vi "DSF.Memory.Pointer.Channel Properties.Write.1D.vi"(7 "count (-1: all)":i64=-1 format="%d elements", 8 "error in (no error)":errorcluster, 9 "buffer in":T1[](array[typedef]) {"count" format="%d elements"; "size" format="%d bytes"; "offset" format="%d bytes"}, 10 "index (0)":u64 format="%d elements", 11 "Channel Properties Pointer in":refnum<class "DSF.Memory.Pointer.Channel Properties.lvclass">) -> (0 "error out":errorcluster, 1 "buffer out":T1[](array[typedef]) {"count" format="%d elements"; "size" format="%d bytes"; "offset" format="%d bytes"}, 2 "index out":u64 format="%d elements", 3 "Channel Properties Pointer out":refnum<class "DSF.Memory.Pointer.Channel Properties.lvclass">)   [LabVIEW 2016, in "DSF.Memory.lvlib" / "DSF.Memory.Pointer.Channel Properties.lvclass"]
uses:
  DSF.Memory.Pointer.Channel Properties.lvclass
  C:/Git/SourceTree/DSF/Source/Classes/Memory.Pointer.Array/DSF.Memory.Pointer.Array.lvclass
  C:/Git/SourceTree/DSF/Source/Submodules/Memory Manager/Source/Classes/Pointer/Memory.Pointer.lvclass
  Typedefs/DSF.Common.Channel Configuration.ctl
  Typedefs/DSF.Common.Data Type.ctl
  Memory.Pointer.Array/DSF.Memory.Pointer.Array.lvclass/DSF.Memory.Pointer.Array.ctl
  Submodules/Memory Manager/Source/Classes/Pointer/Memory.Pointer.lvclass/Memory.Pointer.ctl
  Submodules/Memory Manager/Source/Classes/Pointer/Methods/Memory.Pointer.Errors.vi
  Submodules/Memory Manager/Source/Classes/Pointer/Methods/Memory.Pointer.Errors.Out of Bounds.vi
  Submodules/Memory Manager/Source/Classes/Pointer/Accessors/Get Size.vi
  Submodules/Memory Manager/Source/Submodules/SEH/Source/VIs/Static Error Handling.Source Buffer.Write.String.vi
  Submodules/Memory Manager/Source/Classes/Pointer/Methods/Memory.Pointer.Errors.Write Pointer Size.vi
  Submodules/Memory Manager/Source/Classes/Pointer/Methods/Memory.Pointer.Errors.Create Error.vi
  Submodules/Memory Manager/Source/Submodules/SEH/Source/VIs/Static Error Handling.Source Buffer.Write.Numeric.Scalar.Base10.vi
  Submodules/Memory Manager/Source/Submodules/SEH/Source/VIs/Static Error Handling.Source Buffer.Write.Numeric.Scalar.Base10 (U64).vi
  Submodules/Memory Manager/Source/Submodules/SEH/Source/VIs/Static Error Handling.Error Cluster Constant.vi
  Submodules/Memory Manager/Source/Submodules/SEH/Source/VIs/Static Error Handling.Error Cluster Constant (256B).vi
  Submodules/Memory Manager/Source/Submodules/SEH/Source/VIs/Static Error Handling.Parameters.Status.Set.vi
  Submodules/Memory Manager/Source/Submodules/SEH/Source/VIs/Static Error Handling.Parameters.Code.Set.vi
  Submodules/Memory Manager/Source/Submodules/SEH/Source/VIs/Static Error Handling.Parameters.VI Source.Set.vi
  Submodules/Memory Manager/Source/Constants/Memory.Constants.vi
  Submodules/Memory Manager/Source/Constants/Memory.Constants.Library Name.vi
  Submodules/Memory Manager/Source/Classes/Pointer/Methods/Memory.Pointer.Errors.Get Info.vi
  Memory.Pointer.Array/DSF.Memory.Pointer.Array.lvclass
  Submodules/Memory Manager/Source/Classes/Pointer/Memory.Pointer.lvclass
  DSF.Common.lvlib
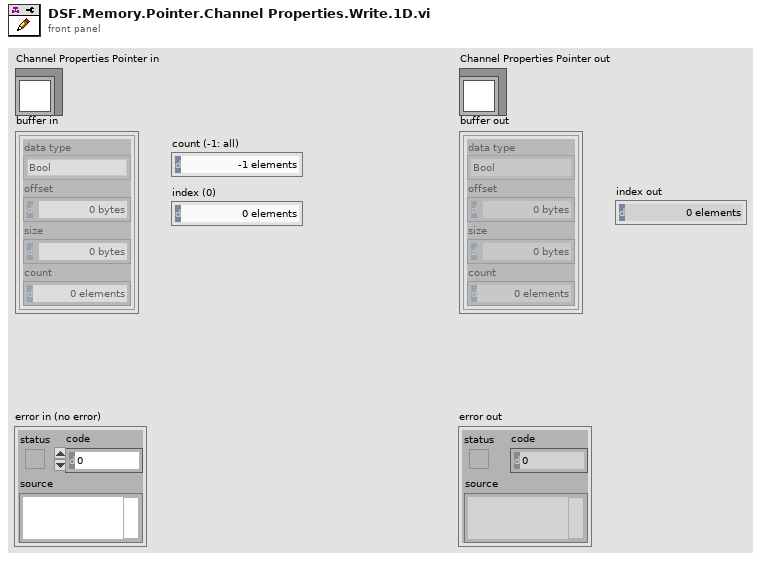
[diagram p1: front panel]
types:
  T1 = typedef "DSF.Common.lvlib/DSF.Common.Channel Configuration.ctl" = cluster{"data type":T2, "offset":u64, "size":u64, "count":u64}
  T2 = typedef "DSF.Common.lvlib/DSF.Common.Data Type.ctl" = enum8{"Bool", "SGL", "DBL", "I8", "I16", "I32", "I64", "U8", "U16", "U32", "U64"}
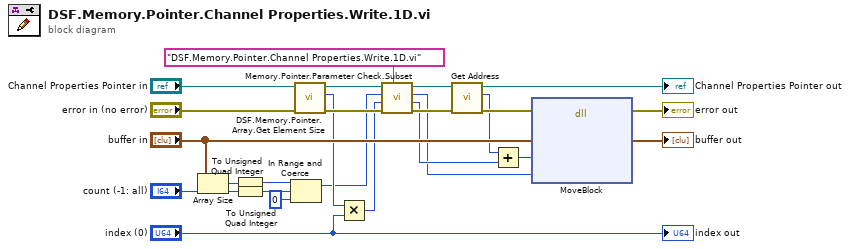
[diagram p0: block diagram]
diagram:
  n1 = Array Size(array="buffer in") -> (size(s)=w7:i32)
  n2 = To Unsigned Quad Integer(1:w7) -> (0:w6:u64)
  n3 = To Unsigned Quad Integer(1:"count (-1: all)") -> (0:w8:u64)
  n4 = In Range and Coerce(upper limit=w6, x=w8, lower limit=u64 0) -> (coerced(x)=w5:u64)  [unwired: 1 out]
  n5 = call "DSF.Memory.Pointer.Array.Get Element Size.vi"("error in (no error)"="error in (no error)", "Array Pointer in"="Channel Properties Pointer in") -> ("error out"=w19:errorcluster, "element size"=w13:u64, "Array Pointer out"=w20:refnum<class "DSF.Memory.Pointer.Channel Properties.lvclass">)  [unwired: 7 in]
  n6 = Multiply(x=w13, y="index (0)") -> (x*y=w12:u64)
  n7 = call "Memory.Pointer.Parameter Check.Subset.vi"("source vi name"="DSF.Memory.Pointer.Channel Properties.Write.1D.vi", "error in (no error)"=w19, "offset (0)"=w12, "length"=w5, "Pointer in"=w20) -> ("error out"=w17:errorcluster, "offset out"=w15:u64, "length"=w14:u64, "Pointer out"=w18:refnum<class "DSF.Memory.Pointer.Channel Properties.lvclass">)  [unwired: 3 in]
  n8 = call "Get Address.vi"("error in (no error)"=w17, "Pointer in"=w18) -> ("error out"=w24:errorcluster, "address"=w22:u64, "Pointer out"=→"Channel Properties Pointer out":refnum<class "DSF.Memory.Pointer.Channel Properties.lvclass">)  [unwired: 7 in]
  n9 = Add(x=w22, y=w15) -> (x+y=w1:u64)
  n10 = dll-call lib="LabVIEW" fn="MoveBlock"(error in=w24, "src"="buffer in", "dst"=w1, "size"=w14) -> (error out=→"error out":errorcluster, "src"=→"buffer out":T1[])  [unwired: 5 in, 1 out]
  "index out" <- "index (0)"
